vi "Array2String.vi"(7 "Use Space":bool, 10 "Array":dbl[](array[numeric])) -> (2 "String":string)   [LabVIEW 2013]
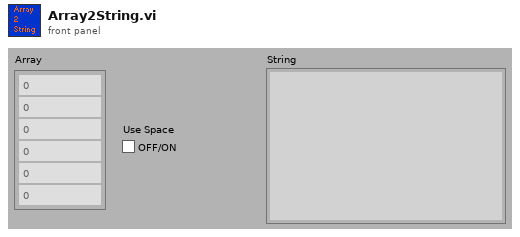
[diagram p1: front panel]
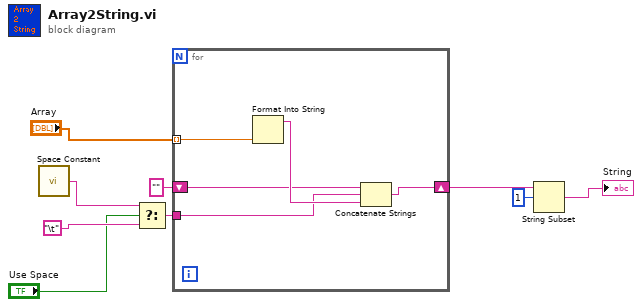
[diagram p0: block diagram]
diagram:
  n1 = call <vilib>:"Space Constant.vi"() -> ("String"=w1:string)
  n2 = Select(t=w1, s="Use Space", f="\t") -> (s? t:f=w4:string)
  n3 = for {
    tunnel: "Array" -> [w14] mode=indexing
    shift-right: [w11] -> w7
    shift-left: "" -> [w12]
    tunnel: w4 -> [w10]
    n4 = Format Into String(w14) -> (resulting string=w13:string)  [unwired: 3 in, 1 out]
    n5 = Concatenate Strings(w12, w10, w13) -> (w11:string)
  }
  n6 = String Subset(string=w7, offset (0)=1) -> (substring=→"String":string)  [unwired: 1 out]
